vi "Set Pre and Post Build Actions.vi"(8 "error in (no error)":errorcluster, 9 "Post Build Action VI":refnum<vi>, 10 "Pre Build Action VI":refnum<vi>, 11 "Build in":refnum<class "NI_AB_API_DLL.lvclass">) -> (0 "error out":errorcluster, 3 "Build out":refnum<class "NI_AB_API_DLL.lvclass">)   [LabVIEW 2020, in "NI_AB_API_DLL.lvclass"]
uses:
  <vilib>/AppBuilder/AB_API/DLL/NI_AB_API_DLL.lvclass
  <vilib>/AppBuilder/AB_API/DLL/NI_AB_API_DLL.lvclass/NI_AB_API_DLL.ctl
  <vilib>/AppBuilder/AB_API/Application/NI_AB_API_Application.lvclass
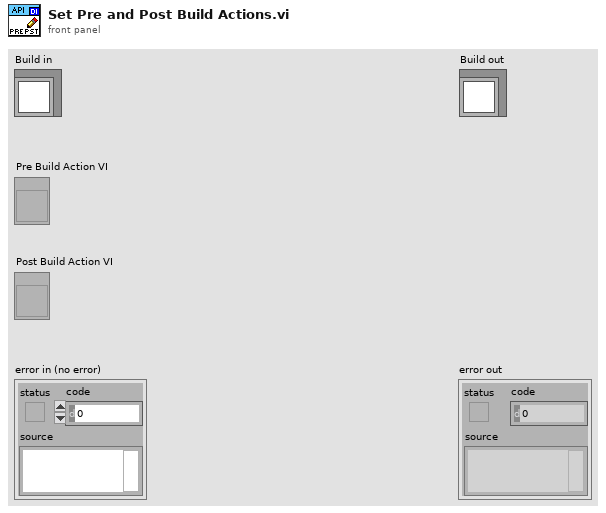
[diagram p1: front panel]
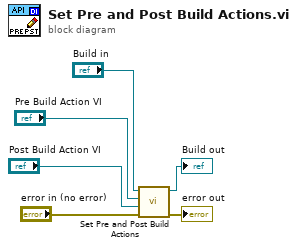
[diagram p0: block diagram]
diagram:
  n1 = call-parent "Set Pre and Post Build Actions.vi"("error in (no error)"="error in (no error)", "Post Build Action VI"="Post Build Action VI", "Pre Build Action VI"="Pre Build Action VI", "Build in"="Build in") -> ("error out"=→"error out":errorcluster, "Build out"=→"Build out":refnum<class "NI_AB_API_DLL.lvclass">)  [unwired: 6 in]
